vi "Teleop.vi"(10 "Match Info":T1={"Autonomous Elapsed Seconds"=0.0, "TeleOp Elapsed Seconds"=0.0, "Disabled Elapsed Seconds"=0.0, "Visited Autonomous"=FALSE, "Visited TeleOp"=FALSE, "Visited Disabled"=FALSE, "Autonomous Settings"={"Autonomous Style"=enum."Independent", "VI Refnum"=refnum}}, 11 "Call Context":T2) -> ()   [LabVIEW 2013]
doc: "This VI is called for each TeleOp packet received from the DS where the robot is not disabled. It is often used to read from the joysticks and update I/O or to update setpoints for timed control loops. It should complete and return within 20 milliseconds or it may miss DS packets."
uses:
  <vilib>/Rock Robotics/WPI/DriverStation/WPI_DriverStationDerivedRobotMode.ctl
  <vilib>/Rock Robotics/WPI/DriverStation/WPI_DriverStationMatch Info.ctl
  Robot Global Data.vi
  <vilib>/Rock Robotics/WPI/Joystick/WPI_JoystickGetSetRefNum.vi
  <vilib>/Rock Robotics/WPI/RobotDrive/WPI_RobotDriveMecanumDrive_Cartesian.vi
  <vilib>/Rock Robotics/WPI/RobotDrive/WPI_RobotDriveGetSetRefNum.vi
panel:
  out "Numeric 1":dbl(slide) scale=0.0..100.0
  out "Boolean 2":bool
  out "Boolean 1":bool
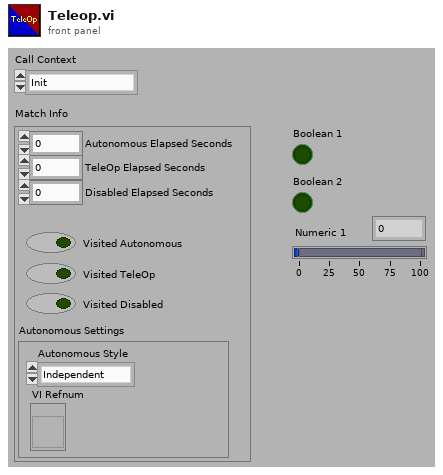
[diagram p1: front panel]
types:
  T1 = typedef "WPI_DriverStationMatch Info.ctl" = cluster{"Autonomous Elapsed Seconds":dbl, "TeleOp Elapsed Seconds":dbl, "Disabled Elapsed Seconds":dbl, "Visited Autonomous":bool, "Visited TeleOp":bool, "Visited Disabled":bool, "Autonomous Settings":cluster{"Autonomous Style":enum16{"Iterative", "Independent"}, "VI Refnum":refnum<vi>}}
  T2 = typedef "WPI_DriverStationDerivedRobotMode.ctl" = enum16{"Init", "Execute", "Stop"}
  T3 = typedef "WPI_JoystickDevRef.ctl" = cluster{"Device":T4}
  T4 = typedef "WPI_JoystickDeviceEnum.ctl" = enum16{"USB 1", "USB 2", "USB 3", "USB 4", "Kinect 1", "Kinect 2"}
  T5 = typedef "WPI_JoystickButtonState.ctl" = cluster{"Button 1":bool, "Button 2":bool, "Button 3":bool, "Button 4":bool, "Button 5":bool, "Button 6":bool, "Button 7":bool, "Button 8":bool, "Button 9":bool, "Button 10":bool, "Button 11":bool, "Button 12":bool}
  T6 = cluster{"axis 1 (x)":dbl, "axis 2 (y)":dbl, "axis 3 (throttle)":dbl, "axis 4":dbl, "axis 5":dbl, "axis 6":dbl}
  T7 = typedef "WPI_RobotDriveDevRef.ctl" = cluster{"DevStatus":errorcluster, "Motors[]":T8[], "Square Inputs":bool, "Max Output":dbl, "Isochronous":bool}
  T8 = typedef "WPI_MotorControlDeviceRef.ctl" = cluster{"DeviceStatus":errorcluster, "Type":enum16{"PWM", "CAN"}, "PWM":cluster{"Digital Module":T9, "PWM Channel":T10, "DeadBand":T11}, "CAN":cluster{"Device Number":u8, "Control Mode":T12, "Semaphore":T13, "Max Vout":dbl}, "Invert":bool, "TransformRef":T14, "InvTransformRef":T14}
  T9 = typedef "FPGA_TypedefDigitalModule.ctl" = enum16{"Digital Module 1", "Digital Module 2"}
  T10 = typedef "FPGA_DIOPWMChannel.ctl" = enum8{"PWM 1", "PWM 2", "PWM 3", "PWM 4", "PWM 5", "PWM 6", "PWM 7", "PWM 8", "PWM 9", "PWM 10", "Invalid"}
  T11 = typedef "WPI_PWMDeadband.ctl" = cluster{"Name":string, "maxPositivePwm":i32, "minPositivePwm":i32, "centerPwm":i32, "maxNegativePwm":i32, "minNegativePwm":i32, "angularRange":u16}
  T12 = typedef "WPI_CANJaguar_ControlMode.ctl" = enum8{"Percent VBus", "Current", "Speed", "Position", "Voltage"}
  T13 = typedef "Semaphore RefNum" = refnum<k1>
  T14 = typedef "WPI_PWMTransform_ConPane.ctl" = refnum<vi>
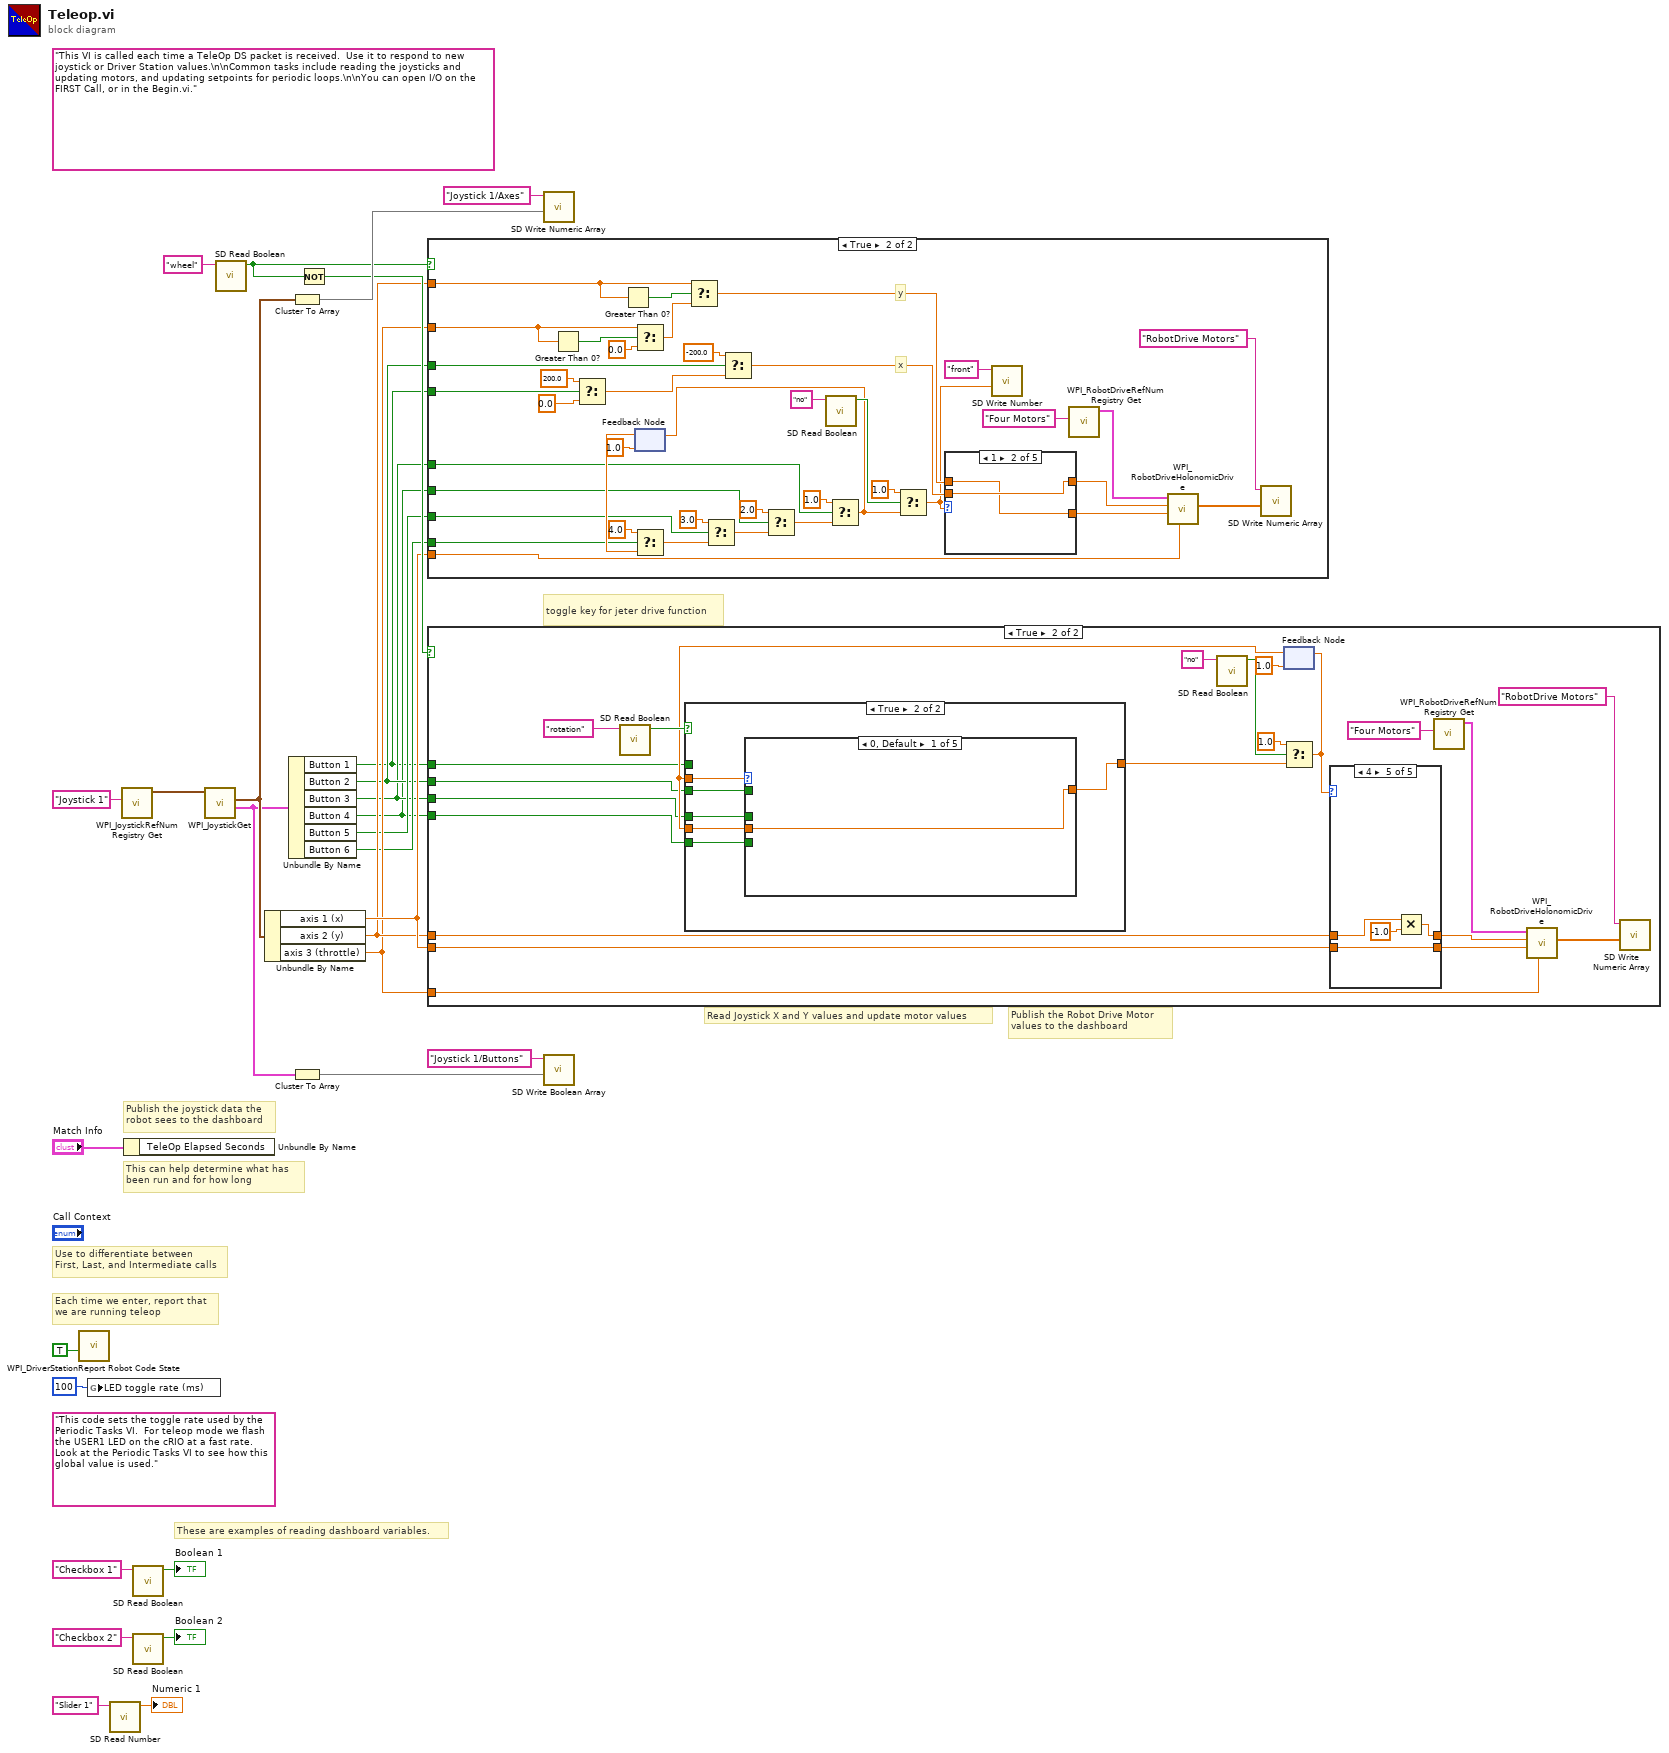
[diagram p0: block diagram]
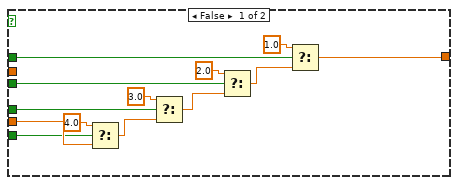
[diagram p3: hidden frame]
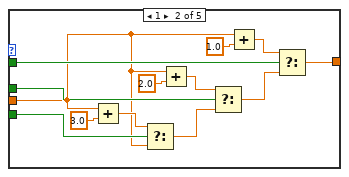
[diagram p4: hidden frame]
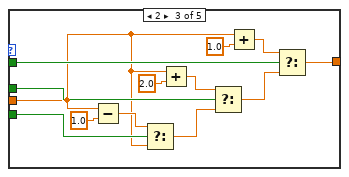
[diagram p5: hidden frame]
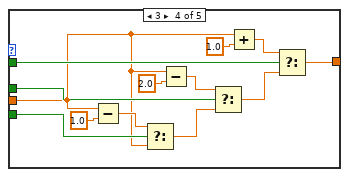
[diagram p6: hidden frame]
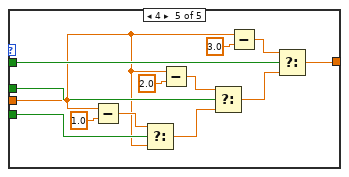
[diagram p7: hidden frame]
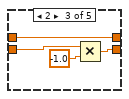
[diagram p10: hidden frame]
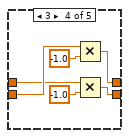
[diagram p11: hidden frame]
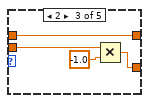
[diagram p14: hidden frame]
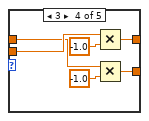
[diagram p15: hidden frame]
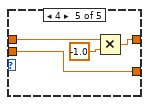
[diagram p16: hidden frame]
diagram:
  (unwired) "This code sets the toggle rate used by the Periodic Tasks VI.  For teleop mode we flash the USER1 LED on the cRIO at a fast rate.  Look at the Periodic Tasks VI to see how this global value is used."
  (unwired) "This VI is called each time a TeleOp DS packet is received.  Use it to respond to new joystick or Driver Station values.\n\nCommon tasks include reading the joysticks and updating motors, and updating setpoints for periodic loops.\n\nYou can open I/O on the FIRST Call, or in the Begin.vi."
  # "Publish the joystick data the\nrobot sees to the dashboard"
  # "toggle key for jeter drive function"
  # "These are examples of reading dashboard variables."
  # "Publish the Robot Drive Motor\nvalues to the dashboard"
  # "Each time we enter, report that\nwe are running teleop"
  # "Use to differentiate between\nFirst, Last, and Intermediate calls"
  # "This can help determine what has\nbeen run and for how long"
  # "Read Joystick X and Y values and update motor values"
  n1 = call <vilib>:"WPI_DriverStationReport Robot Code State.vi"("TeleOp"=TRUE ("Autonomous")) -> ()  [unwired: 10 in, 1 out]
  n2 = global write "Robot Global Data.vi" "LED toggle rate (ms)"(u32 100 ("LED ms toggle rate")) -> ()
  n3 = call <vilib>:"SD Read Number.vi"("Name"="Slider 1" ("refnum name")) -> ("Numeric"=→"Numeric 1":dbl)  [unwired: 8 in, 2 out]
  n4 = call <vilib>:"WPI_JoystickRefNum Registry Get.vi"("refnum name"="Joystick 1") -> ("JoystickDevRef"=w27:T3)  [unwired: 1 in, 9 out]
  n5 = Unbundle By Name("Match Info") -> ()  [unwired: 1 out]
  n6 = call <vilib>:"SD Read Boolean.vi"("Name"="Checkbox 1" ("refnum name")) -> ("Boolean"=→"Boolean 1":bool)  [unwired: 8 in, 2 out]
  n7 = call <vilib>:"SD Read Boolean.vi"("Name"="Checkbox 2" ("refnum name")) -> ("Boolean"=→"Boolean 2":bool)  [unwired: 8 in, 2 out]
  n8 = call <vilib>:"WPI_JoystickGet.vi"("JoystickDevRef"=w27) -> ("Buttons"=w15:T5, "Axes"=w24:T6)  [unwired: 1 in, 4 out]
  n9 = call <vilib>:"SD Read Boolean.vi"("Name"="wheel") -> ("Boolean"=w14:bool)  [unwired: 8 in, 2 out]
  n10 = Unbundle By Name(w24) -> ("axis 1 (x)"=w9:dbl, "axis 2 (y)"=w8:dbl, "axis 3 (throttle)"=w7:dbl)
  n11 = Unbundle By Name(w15) -> ("Button 1"=w1:bool, "Button 2"=w4:bool, "Button 3"=w3:bool, "Button 4"=w2:bool, "Button 5"=w6:bool, "Button 6"=w5:bool)
  n12 = Cluster To Array(cluster=w24) -> (array=w23:dbl[])
  n13 = Cluster To Array(cluster=w15) -> (array=w10:bool[])
  n14 = Not(x=w14) -> (.not. x?=w13:bool)
  n15 = case shown="True" w14 {
    tunnel: w1 -> [_ w65]
    tunnel: w4 -> [_ w64]
    tunnel: w9 -> [_ w60]
    tunnel: w7 -> [_ w59]
    tunnel: w8 -> [_ w49]
    tunnel: w3 -> [_ w39]
    tunnel: w2 -> [_ w38]
    tunnel: w6 -> [_ w37]
    tunnel: w5 -> [_ w36]
    frame False {
    }
    frame True {
      # "y"
      # "x"
      n16 = Greater Than 0?(x=w59) -> (x > 0?=w56:bool)
      n17 = Select(t=200.0, s=w65, f=0.0) -> (s? t:f=w63:dbl)
      n18 = Greater Than 0?(x=w49) -> (x > 0?=w57:bool)
      n19 = Select(t=w59, s=w56, f=0.0) -> (s? t:f=w58:dbl)
      n20 = feedback #1(1.0) -> (w41:dbl)
      n21 = Select(t=4.0, s=w36, f=w41) -> (s? t:f=w43:dbl)
      n22 = Select(t=w49, s=w57, f=w58) -> (s? t:f=w50:dbl)
      n23 = Select(t=3.0, s=w37, f=w43) -> (s? t:f=w44:dbl)
      n24 = Select(t=-200.0, s=w64, f=w63) -> (s? t:f=w53:dbl)
      n25 = Select(t=2.0, s=w38, f=w44) -> (s? t:f=w45:dbl)
      n26 = call <vilib>:"SD Read Boolean.vi"("Name"="no") -> ("Boolean"=w47:bool)  [unwired: 8 in, 2 out]
      n27 = Select(t=1.0, s=w39, f=w45) -> (s? t:f=w42:dbl)
      n28 = feedback-in #1(w42) -> ()
      n29 = Select(t=1.0, s=w47, f=w42) -> (s? t:f=w35:dbl)
      n30 = case shown="1" w35 {
        tunnel: w53 -> [w70 w73 w76 w83 w84]
        tunnel: [w71 w73 w77 w78 w85] -> w52
        tunnel: [w70 w72 w75 w79 w84] -> w51
        tunnel: w50 -> [w71 w72 w77 w80 w86]
        frame 0, Default {
        }
        frame 1 {
        }
        frame 2 {
          n31 = Multiply(x=w76, y=-1.0) -> (x*y=w75:dbl)
        }
        frame 3 {
          n32 = Multiply(x=w83, y=-1.0) -> (x*y=w78:dbl)
          n33 = Multiply(x=w80, y=-1.0) -> (x*y=w79:dbl)
        }
        frame 4 {
          n34 = Multiply(x=w86, y=-1.0) -> (x*y=w85:dbl)
        }
      }
      n35 = call <vilib>:"SD Write Number.vi"("Numeric"=w35, "Name"="front") -> ()  [unwired: 8 in, 2 out]
      n36 = call <vilib>:"WPI_RobotDriveRefNum Registry Get.vi"("refnum name"="Four Motors") -> ("RobotDriveDevRef"=w68:T7)  [unwired: 1 in, 9 out]
      n37 = call-poly <vilib>:"WPI_RobotDriveHolonomicDrive.vi"("Rotation"=w60, "Y"=w51, "X"=w52, "RobotDriveDevRef"=w68) -> ("Motor Values"=w66:dbl[])  [unwired: 5 in, 2 out]
      n38 = call <vilib>:"SD Write Numeric Array.vi"("Numeric Array"=w66, "Name"="RobotDrive Motors") -> ()  [unwired: 8 in, 2 out]
    }
  }
  n39 = case shown="True" w13 {
    tunnel: w9 -> [_ w100]
    tunnel: w8 -> [_ w102]
    tunnel: w7 -> [_ w105]
    tunnel: w4 -> [_ w93]
    tunnel: w3 -> [_ w92]
    tunnel: w2 -> [_ w91]
    tunnel: w1 -> [_ w88]
    frame False {
    }
    frame True {
      n40 = call <vilib>:"SD Read Boolean.vi"("Name"="rotation") -> ("Boolean"=w99:bool)  [unwired: 8 in, 2 out]
      n41 = call <vilib>:"SD Read Boolean.vi"("Name"="no") -> ("Boolean"=w89:bool)  [unwired: 8 in, 2 out]
      n42 = feedback #2(1.0 ("t")) -> (w95:dbl)
      n43 = case shown="True" w99 {
        tunnel: w95 -> [_ w128]
        tunnel: w95 -> [w118 w127]
        tunnel: [w122 w126] -> w94
        tunnel: w93 -> [w116 w125]
        tunnel: w92 -> [w115 w124]
        tunnel: w91 -> [w114 w123]
        tunnel: w88 -> [w117 _]
        frame False {
          n44 = Select(t=4.0, s=w114, f=w118) -> (s? t:f=w119:dbl)
          n45 = Select(t=3.0, s=w115, f=w119) -> (s? t:f=w120:dbl)
          n46 = Select(t=2.0, s=w116, f=w120) -> (s? t:f=w121:dbl)
          n47 = Select(t=1.0, s=w117, f=w121) -> (s? t:f=w122:dbl)
        }
        frame True {
          n48 = case shown="0, Default" w128 {
            tunnel: w127 -> [w129 w134 w144 w158 w173]
            tunnel: [w129 w140 w155 w168 w181] -> w126
            tunnel: w125 -> [_ w139 w152 w162 w175]
            tunnel: w124 -> [_ w138 w151 w163 w176]
            tunnel: w123 -> [_ w137 w150 w164 w177]
            frame 0, Default {
            }
            frame 1 {
              n49 = Add(x=w134, y=3.0) -> (x+y=w135:dbl)
              n50 = Select(t=w135, s=w137, f=w134) -> (s? t:f=w142:dbl)
              n51 = Add(x=w134, y=2.0) -> (x+y=w132:dbl)
              n52 = Select(t=w132, s=w138, f=w142) -> (s? t:f=w141:dbl)
              n53 = Add(x=w134, y=1.0) -> (x+y=w136:dbl)
              n54 = Select(t=w136, s=w139, f=w141) -> (s? t:f=w140:dbl)
            }
            frame 2 {
              n55 = Subtract(x=w144, y=1.0) -> (x-y=w149:dbl)
              n56 = Select(t=w149, s=w150, f=w144) -> (s? t:f=w154:dbl)
              n57 = Add(x=w144, y=2.0) -> (x+y=w147:dbl)
              n58 = Select(t=w147, s=w151, f=w154) -> (s? t:f=w153:dbl)
              n59 = Add(x=w144, y=1.0) -> (x+y=w145:dbl)
              n60 = Select(t=w145, s=w152, f=w153) -> (s? t:f=w155:dbl)
            }
            frame 3 {
              n61 = Subtract(x=w158, y=1.0) -> (x-y=w165:dbl)
              n62 = Select(t=w165, s=w164, f=w158) -> (s? t:f=w166:dbl)
              n63 = Subtract(x=w158, y=2.0) -> (x-y=w159:dbl)
              n64 = Select(t=w159, s=w163, f=w166) -> (s? t:f=w167:dbl)
              n65 = Add(x=w158, y=1.0) -> (x+y=w157:dbl)
              n66 = Select(t=w157, s=w162, f=w167) -> (s? t:f=w168:dbl)
            }
            frame 4 {
              n67 = Subtract(x=w173, y=1.0) -> (x-y=w178:dbl)
              n68 = Select(t=w178, s=w177, f=w173) -> (s? t:f=w179:dbl)
              n69 = Subtract(x=w173, y=2.0) -> (x-y=w172:dbl)
              n70 = Select(t=w172, s=w176, f=w179) -> (s? t:f=w180:dbl)
              n71 = Subtract(x=w173, y=3.0) -> (x-y=w171:dbl)
              n72 = Select(t=w171, s=w175, f=w180) -> (s? t:f=w181:dbl)
            }
          }
        }
      }
      n73 = Select(t=1.0, s=w89, f=w94) -> (s? t:f=w97:dbl)
      n74 = feedback-in #2(w97) -> ()
      n75 = case shown="4" w97 {
        tunnel: [w183 w185 w189 w193 w196] -> w103
        tunnel: w102 -> [w182 w184 w189 w190 w197]
        tunnel: [w182 w184 w186 w192 w199] -> w101
        tunnel: w100 -> [w183 w185 w187 w191 w199]
        frame 0, Default {
        }
        frame 1 {
        }
        frame 2 {
          n76 = Multiply(x=w187, y=-1.0) -> (x*y=w186:dbl)
        }
        frame 3 {
          n77 = Multiply(x=w191, y=-1.0) -> (x*y=w193:dbl)
          n78 = Multiply(x=w190, y=-1.0) -> (x*y=w192:dbl)
        }
        frame 4 {
          n79 = Multiply(x=w197, y=-1.0) -> (x*y=w196:dbl)
        }
      }
      n80 = call <vilib>:"WPI_RobotDriveRefNum Registry Get.vi"("refnum name"="Four Motors") -> ("RobotDriveDevRef"=w108:T7)  [unwired: 1 in, 9 out]
      n81 = call-poly <vilib>:"WPI_RobotDriveHolonomicDrive.vi"("Rotation"=w105, "Y"=w101, "X"=w103, "RobotDriveDevRef"=w108) -> ("Motor Values"=w106:dbl[])  [unwired: 5 in, 2 out]
      n82 = call <vilib>:"SD Write Numeric Array.vi"("Numeric Array"=w106, "Name"="RobotDrive Motors") -> ()  [unwired: 8 in, 2 out]
    }
  }
  n83 = call <vilib>:"SD Write Numeric Array.vi"("Numeric Array"=w23, "Name"="Joystick 1/Axes") -> ()  [unwired: 8 in, 2 out]
  n84 = call <vilib>:"SD Write Boolean Array.vi"("Boolean Array"=w10, "Name"="Joystick 1/Buttons") -> ()  [unwired: 8 in, 2 out]
